vi "Check if Panther Logs Enabled.vi"() -> (3 "PantherLogs Enabled?":bool)   [LabVIEW 2016, in "PantherLAB_Log.lvlib"]
uses:
  PantherLAB_Log.lvlib
  <resource>/dialog/lvconfig.llb/LV Config Read Boolean.vi
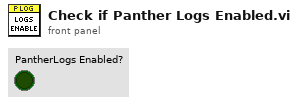
[diagram p1: front panel]
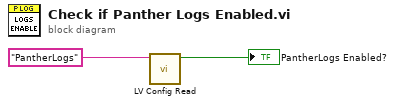
[diagram p0: block diagram]
diagram:
  n1 = call-poly <resource>:"LV Config Read.vi"("key"="PantherLogs") -> ("value"=→"PantherLogs Enabled?":bool)  [unwired: 4 in, 2 out]
